vi "PmSetRegion.vi"(8 "error in (no error)":errorcluster, 10 "Exposure (ms)":dbl, 11 "reference in":refnum<k24>) -> (0 "error out":errorcluster, 3 "reference out":refnum<k24>)   [LabVIEW 2022 SP3, in "Photometrics Camera.lvlib"]
uses:
  Photometrics Camera.lvlib
  C:/FlashGordon/Development/dll/PVCamNET.dll
  dll/PVCamNET.dll
panel:
  out "Width":u16
  out "Height":u16
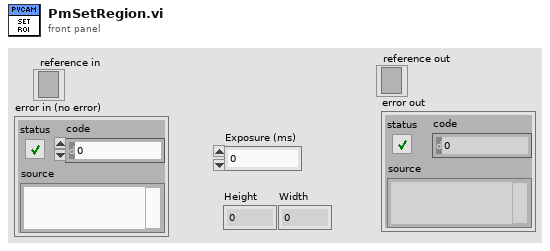
[diagram p1: front panel]
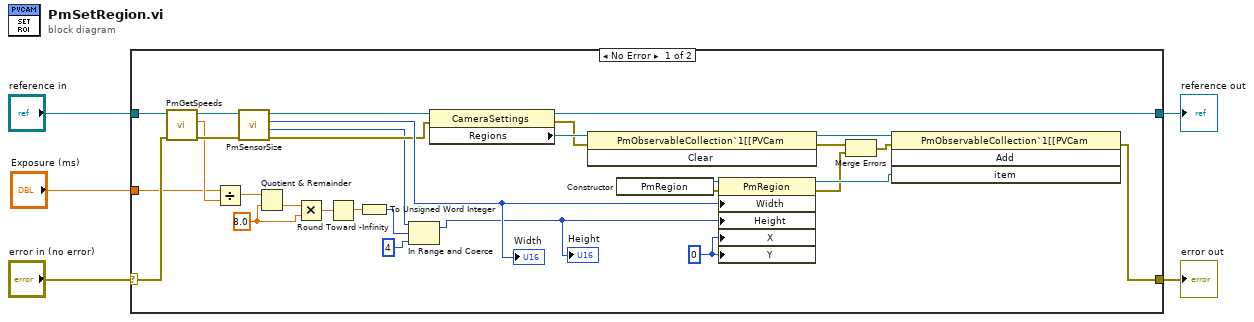
[diagram p0: block diagram]
diagram:
  n1 = case shown="No Error" "error in (no error)" {
    selector: "error in (no error)" -> [w20 w36]
    tunnel: "reference in" -> [w21 w37]
    tunnel: [w28 w36] -> w3
    tunnel: [w27 w37] -> w2
    tunnel: "Exposure (ms)" -> [w13 _]
    frame No Error {
      w10 = 8.0 ("y")
      w31 = u16 0 ("X")
      n2 = call "PmGetSpeeds.vi"("error in (no error)"=w20, "reference in"=w21) -> ("error out"=w22:errorcluster, "ScanLineTimeMs"=w14:dbl, "reference out"=w25:refnum<k24>)  [unwired: 7 in]
      n3 = Divide(x=w13, y=w14) -> (x/y=w9:dbl)
      n4 = call "PmSensorSize.vi"("error in (no error)"=w22, "reference"=w25) -> ("error out"=w23:errorcluster, "Height"=w19:u16, "Width"=w26:u16, "reference 2"=w24:refnum<k24>)  [unwired: 6 in]
      "Width" <- w26
      n5 = Quotient & Remainder(x=w9, y=w10) -> (floor(x/y)=w11:dbl)  [unwired: 1 out]
      n6 = Multiply(x=w11, y=w10) -> (x*y=w12:dbl)
      n7 = Round Toward -Infinity(1:w12) -> (0:w8:dbl)
      n8 = To Unsigned Word Integer(number=w8) -> (unsigned 16bit integer=w7:u16)
      n9 = In Range and Coerce(upper limit=w19, x=w7, lower limit=u16 4) -> (coerced(x)=w6:u16)  [unwired: 1 out]
      "Height" <- w6
      n10 = property class="CameraSettings"(reference=w24, error in=w23) -> (reference out=w27:refnum<k24>, error out=w29:errorcluster, "Regions"=w30:refnum<k24>)
      n11 = invoke class="PmObservableCollection`1[[PVCam" method="Clear"(reference=w30, error in=w29) -> (reference out=w34:refnum<k24>, error out=w16:errorcluster)  [unwired: 1 in, 1 out]
      n12 = constructor class="PmRegion"() -> (reference out=w33:refnum<k24>, error out=w32:errorcluster)  [unwired: 3 in, 1 out]
      n13 = property class="PmRegion"(reference=w33, error in=w32, "Width"=w26, "Height"=w6, "X"=w31, "Y"=w31) -> (reference out=w35:refnum<k24>, error out=w15:errorcluster)
      n14 = Merge Errors(w16, w15) -> (w17:errorcluster)
      n15 = invoke class="PmObservableCollection`1[[PVCam" method="Add"(reference=w34, error in=w17, "item"=w35) -> (error out=w28:errorcluster)  [unwired: 1 in, 3 out]
    }
    frame Error {
    }
  }
  "reference out" <- w2
  "error out" <- w3
